vi "JAUS Dumb Test.vi"() -> ()   [LabVIEW 2009]
uses:
  UDP Lib/UDP Network Location.ctl
panel:
  in  "Source ID (80-95)":u16=253
  out "HB":bool
  out "Output (Hex)":string
  out "Output (ASCII)":string
  out "Sender":T1
  in  "stop":bool
  in  "Local Port":u16=3794
  in  "Destination Location":T1={"IP Address"="24.42.140.203", "Port"=3794}
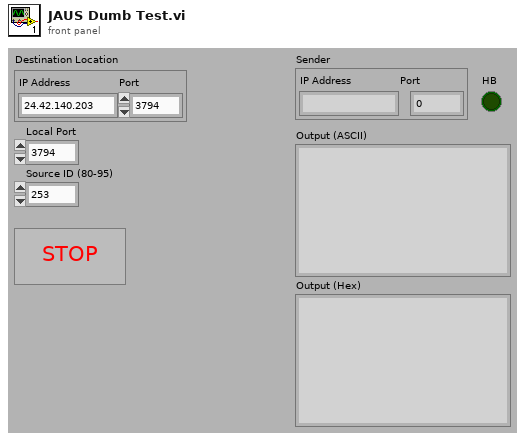
[diagram p1: front panel]
types:
  T1 = typedef "UDP Network Location.ctl" = cluster{"IP Address":string, "Port":u16}
  T2 = typedef "UDP Base.ctl" = cluster{"UDP Session":refnum<k16>, "UDP Socket Params":T3}
  T3 = typedef "UDP Socket Params.ctl" = cluster{"Local Port":u16, "Read Timeout":i32, "Write Timeout":i32}
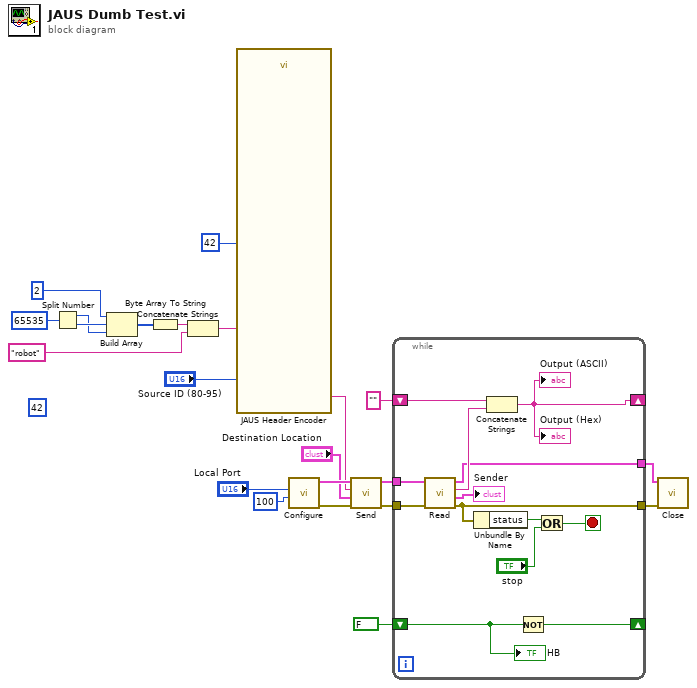
[diagram p0: block diagram]
diagram:
  (unwired) u32 42 ("Destination ID (48-79)")
  n1 = Split Number(x=u16 65535 ("Destination ID (48-79)")) -> (hi(x)=w3:u8, lo(x)=w4:u8)
  n2 = Build Array(u8 2 ("Destination ID (48-79)"), w4, w3) -> (w7:u8[])
  n3 = Byte Array To String(unsigned byte array=w7) -> (string=w8:string)
  n4 = Concatenate Strings(w8, "robot" ("string")) -> (w2:string)
  n5 = call "JAUS Header Encoder.vi"("Payload"=w2, "Source ID (80-95)"="Source ID (80-95)", "Destination ID (48-79)"=u32 42) -> ("Encoded JAUS Message"=w12:string)  [unwired: 12 in]
  n6 = call "Configure.vi"("Read Timeout"=100, "Local Port"="Local Port") -> ("error out"=w21:errorcluster, "UDP Base out"=w22:T2)  [unwired: 8 in]
  n7 = call "Send.vi"("error in (no error)"=w21, "Destination Location"="Destination Location", "Send Data"=w12, "UDP Base in"=w22) -> ("error out"=w16:errorcluster, "UDP Base out"=w17:T2)  [unwired: 5 in, 1 out]
  n8 = while {
    tunnel: w17 -> [w35]
    tunnel: w16 -> [w34]
    shift-right: [w25] -> _
    shift-left: "" -> [w32]
    tunnel: [w31] -> w14
    tunnel: [w26] -> w13
    shift-right: [w23] -> _
    shift-left: FALSE ("HB") -> [w24]
    stop <- w28 stop-if-true
    n9 = call "Read.vi"("error in (no error)"=w34, "UDP Base in"=w35) -> ("error out"=w26:errorcluster, "Network Location"=→"Sender":T1, "Receive Data"=w33:string, "UDP Base out"=w31:T2)  [unwired: 4 in, 2 out]
    n10 = Unbundle By Name(w26) -> ("status"=w30:bool)
    n11 = Concatenate Strings(w32, w33) -> (w25:string)
    "Output (ASCII)" <- w25
    "Output (Hex)" <- w25
    n12 = Not(x=w24) -> (.not. x?=w23:bool)
    n13 = Or(x=w30, y="stop") -> (x .or. y?=w28:bool)
    "HB" <- w24
  }
  n14 = call "Close.vi"("error in (no error)"=w13, "Cluster of class private data"=w14) -> ()  [unwired: 9 in, 1 out]
